vi "KE622x -- 2182 -A Get Digital Filter State.vi"(0 "622x Resource In":refnum<visa-resource-name>, 1 "Check For SCPI Errors? (T)":bool=TRUE, 11 "error in (no error)":errorcluster) -> (4 "622x Resource Out (dupl)":refnum<visa-resource-name>, 8 "Digital Filter Enabled?":bool, 15 "error out":errorcluster)   [LabVIEW 2019, in "Keithley 622x.lvlib"]
uses:
  Keithley 622x.lvlib
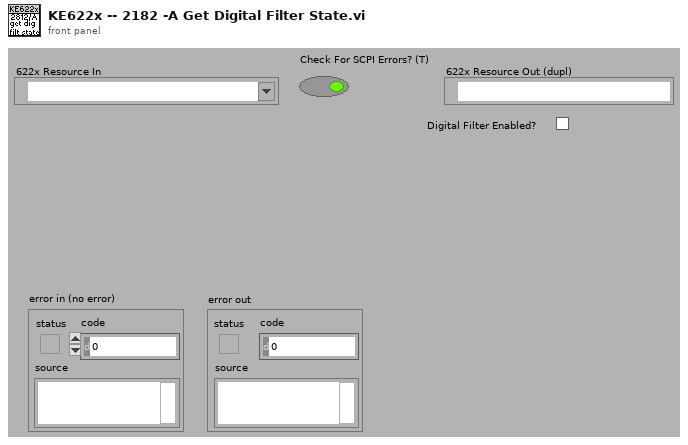
[diagram p1: front panel]
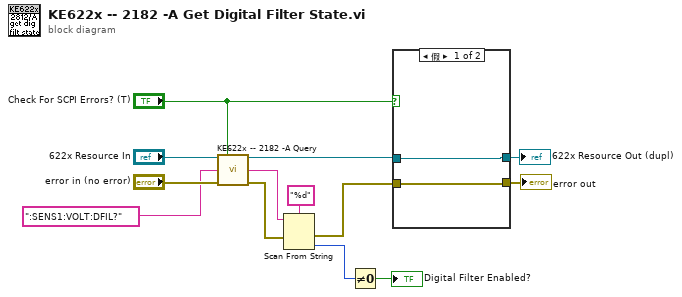
[diagram p0: block diagram]
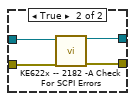
[diagram p2: hidden frame]
diagram:
  n1 = call "KE622x -- 2182 -A Query.vi"("622x Resource In"="622x Resource In", "Check For SCPI Errors? (T)"="Check For SCPI Errors? (T)", "2182-A Write String"=":SENS1:VOLT:DFIL?", "error in (no error)"="error in (no error)") -> ("622x Resource Out (dupl)"=w7:refnum<visa-resource-name>, "2182-A Reponse String"=w8:string, "error out"=w10:errorcluster)  [unwired: 9 in]
  n2 = Scan From String(format string="%d", input string=w8, error in=w10) -> (error out=w6:errorcluster, output 1=w2:i32)  [unwired: 2 in, 2 out]
  n3 = Not Equal To 0?(x=w2) -> (x != 0?=→"Digital Filter Enabled?":bool)
  n4 = case shown="假" "Check For SCPI Errors? (T)" {
    tunnel: w7 -> [w15 w19]
    tunnel: w6 -> [w14 w18]
    tunnel: [w15 w17] -> w4
    tunnel: [w14 w16] -> w3
    frame False {
    }
    frame True {
      n5 = call "KE622x -- 2182 -A Check For SCPI Errors.vi"("VISA Resource In"=w19, "error in (no error)"=w18) -> ("VISA Resource Out (dupl)"=w17:refnum<visa-resource-name>, "error out"=w16:errorcluster)  [unwired: 10 in, 2 out]
    }
  }
  "622x Resource Out (dupl)" <- w4
  "error out" <- w3
